vi "DrawSnake.vi"(8 "error in (no error)":errorcluster, 11 "Snake in":refnum<class "Snake.lvclass">) -> (0 "error out":errorcluster, 3 "Snake out":refnum<class "Snake.lvclass">)   [LabVIEW 2019, in "RT_Game.lvlib" / "Snake.lvclass"]
uses:
  Snake.lvclass
  C:/Users/FreshBob/Dropbox/VIs/myRIO_VGA/Classes/Game/Game.lvclass
  Snake.lvclass/Snake.ctl
  Game/Game.lvclass
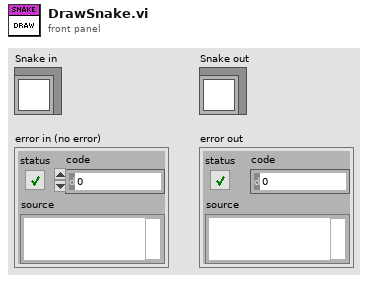
[diagram p1: front panel]
types:
  T1 = typedef "RT_Game.lvlib/Game.lvclass/Coordinate.ctl" = cluster{"x":i16, "y":i16}
  T2 = typedef "RT_Game.lvlib/Snake.lvclass/CoordinateData.ctl" = cluster{"Coordinate":T1, "TileCodes":T3}
  T3 = typedef "RT_Game.lvlib/Game.lvclass/TileCodes.ctl" = enum16{"line_vert", "line_hor", "line_rightup", "line_rightdown", "line_leftup", "line_leftdown", "bg1", "bg2", "bg3", "bg4", "bg5", "bg6", "bg7"}
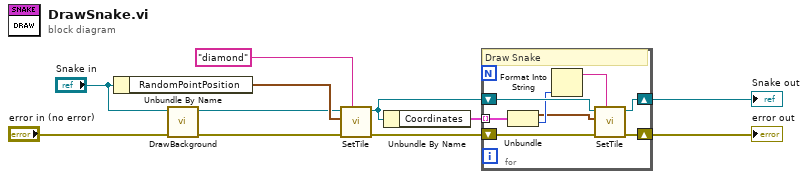
[diagram p0: block diagram]
diagram:
  n1 = Unbundle By Name("Snake in") -> ("RandomPointPosition"=w7:T1)
  n2 = call "DrawBackground.vi"("error in (no error)"="error in (no error)", "Snake in"="Snake in") -> ("error out"=w2:errorcluster, "Snake out"=w4:refnum<class "Snake.lvclass">)  [unwired: 8 in]
  n3 = call "SetTile.vi"("TileCode"="diamond", "error in (no error)"=w2, "Coordinates"=w7, "Game in"=w4) -> ("error out"=w6:errorcluster, "Game out"=w1:refnum<class "Snake.lvclass">)  [unwired: 6 in]
  n4 = Unbundle By Name(w1) -> ("Coordinates"=w11:T2[])
  n5 = for {
    shift-right: [w18] -> w9
    shift-left: w6 -> [w19]
    shift-right: [w16] -> w10
    shift-left: w1 -> [w17]
    tunnel: w11 -> [w15] mode=indexing
    # "Draw Snake"
    n6 = Unbundle(w15) -> ("Coordinate"=w12:T1, "TileCodes"=w13:T3)
    n7 = Format Into String(w13) -> (resulting string=w14:string)  [unwired: 3 in, 1 out]
    n8 = call "SetTile.vi"("TileCode"=w14, "error in (no error)"=w19, "Coordinates"=w12, "Game in"=w17) -> ("error out"=w18:errorcluster, "Game out"=w16:refnum<class "Snake.lvclass">)  [unwired: 6 in]
  }
  "Snake out" <- w10
  "error out" <- w9
